vi "Read_Data_Coils.vi"(8 "error in (no error)":errorcluster, 11 "Device in":refnum<class "RS232_Device.lvclass">) -> (0 "error out":errorcluster, 2 "Discrete Inputs":bool[](array[boolean]), 3 "Device out":refnum<class "RS232_Device.lvclass">)   [LabVIEW 2023, in "RS232_Device.lvclass"]
uses:
  RS232_Device.lvclass
  D:/SamparkProdLine/subVIs/DAQ Device/Modbus_Device/DAQ_Device.lvclass
  RS232_Device.lvclass/RS232_Device.ctl
panel:
  out "resulting string":string
  out "Response":string
  out "return count":u32
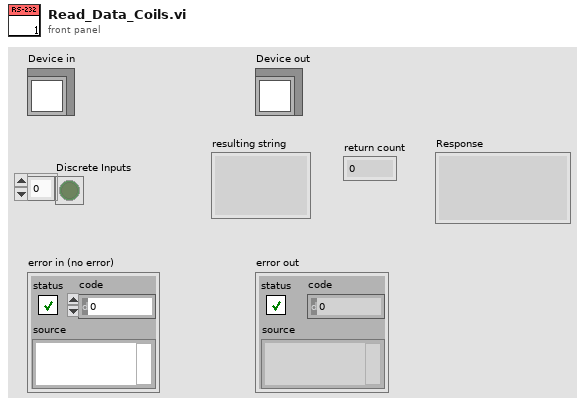
[diagram p1: front panel]
types:
  T1 = typedef "DAQ Device_IO ChannelsData.ctl" = cluster{"#DigitalInputs":u16, "StartAddress_DI":u16, "#DigitalOutputs":u16, "StartAddress_DO":u16, "#AnalogInputs":u16, "StartAddress_AI":u16, "#AnalogOutputs":u16, "StartAddress_AO":u16, "Coil_ReadData":bool[], "Coil_WriteData":bool[], "AI_Data":u16[], "AO_Data":u16[]}
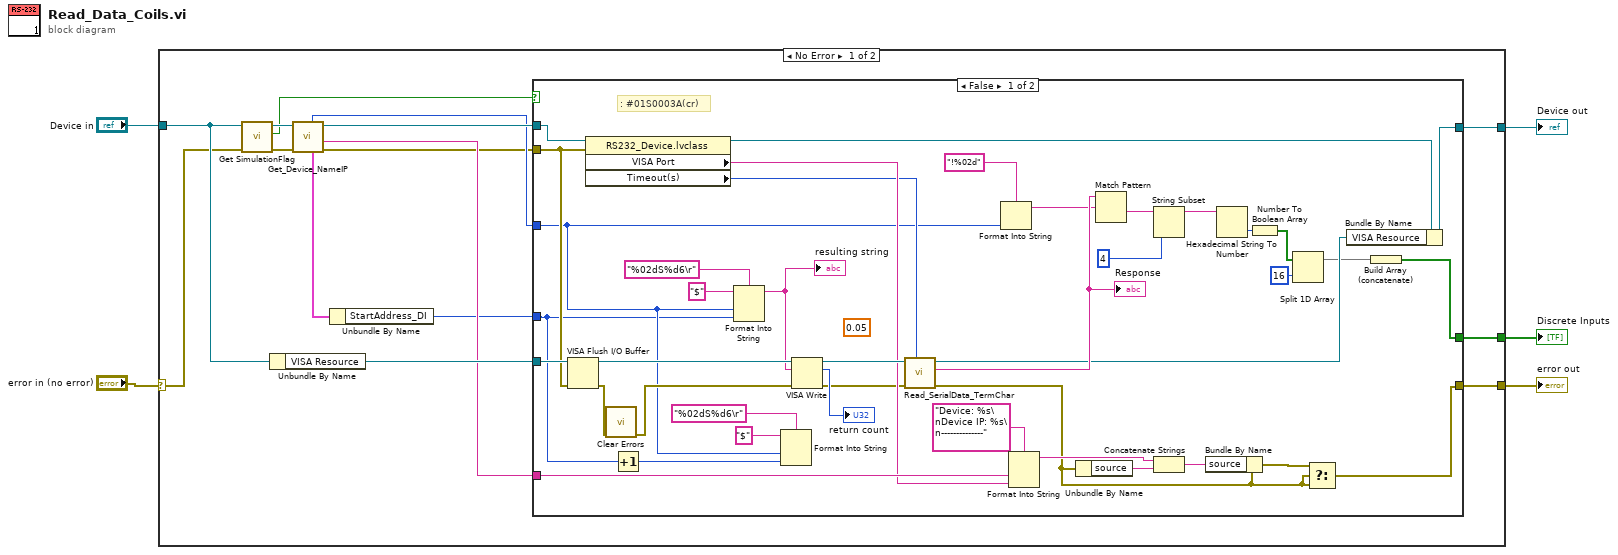
[diagram p0: block diagram]
diagram:
  n1 = case shown="No Error" "error in (no error)" {
    selector: "error in (no error)" -> [w8 w65]
    tunnel: [w19 w65] -> w1
    tunnel: [w20 w64] -> w2
    tunnel: "Device in" -> [w12 w64]
    tunnel: [w17 _] -> w3
    frame No Error {
      n2 = call-dynamic "Get SimulationFlag.vi"("error in (no error)"=w8, "Device in"=w12) -> ("error out"=w16:errorcluster, "Simulation?"=w9:bool, "Device out"=w13:refnum<class "RS232_Device.lvclass">)  [unwired: 7 in]
      n3 = Unbundle By Name(w12) -> ("VISA Resource"=w18:refnum<visa-resource-name>)
      n4 = call-dynamic "Get_Device_NameIP.vi"("error in (no error)"=w16, "Device in"=w13) -> ("error out"=w7:errorcluster, "Device Name"=w10:string, "Device out"=w14:refnum<class "RS232_Device.lvclass">, "IO Channels"=w15:T1, "Unit ID"=w11:u8)  [unwired: 4 in, 1 out]
      n5 = Unbundle By Name(w15) -> ("StartAddress_DI"=w6:u16)
      n6 = case shown="False" w9 {
        tunnel: [w61 w63] -> w20
        tunnel: [w60 w62] -> w19
        tunnel: w18 -> [w59 _]
        tunnel: w14 -> [w41 w63]
        tunnel: w10 -> [w58 _]
        tunnel: [w23 _] -> w17
        tunnel: w11 -> [w30 _]
        tunnel: w6 -> [w29 _]
        tunnel: w7 -> [w40 w62]
        frame False {
          (unwired) 0.05 ("Delay Time (s)")
          # ": #01S0003A(cr)"
          n7 = VISA Flush I/O Buffer(VISA resource name=w59, error in (no error)=w40) -> (VISA resource name out=w52:refnum<visa-resource-name>, error out=w51:errorcluster)  [unwired: 1 in]
          n8 = property class="RS232_Device.lvclass"(reference=w41, error in=w40) -> (reference out=w42:refnum<class "RS232_Device.lvclass">, "VISA Port"=w39:string, "Timeout(s)"=w33:i32)  [unwired: 1 out]
          n9 = call <vilib>:"Clear Errors.vi"("error in (no error)"=w51) -> ("error out"=w50:errorcluster)  [unwired: 5 in, 1 out]
          n10 = Increment(x=w29) -> (x+1=w28:u16)
          n11 = Format Into String(format string="%02dS%d6\r", initial string="$", w30, w29) -> (resulting string=w44:string)  [unwired: 1 in, 1 out]
          "resulting string" <- w44
          n12 = Format Into String(format string="%02dS%d6\r", initial string="$", w30, w28) -> ()  [unwired: 1 in, 2 out]
          n13 = VISA Write(VISA resource name=w52, write buffer=w44, error in (no error)=w50) -> (VISA resource name out=w49:refnum<visa-resource-name>, return count=→"return count":u32, error out=w35:errorcluster)
          n14 = call "Read_SerialData_TermChar.vi"("timeout (50ms)"=w33, "error in (no error)"=w35, "VISA Refnum in"=w49) -> ("error out"=w48:errorcluster, "StringData"=w37:string, "VISA Refnum out"=w34:refnum<visa-resource-name>)  [unwired: 6 in]
          "Response" <- w37
          n15 = Format Into String(format string="!%02d" ("regular expression"), w30) -> (resulting string=w27:string)  [unwired: 2 in, 1 out]
          n16 = Format Into String(format string="Device: %s\nDevice IP: %s\n--------------", w58, w39) -> (resulting string=w54:string)  [unwired: 2 in, 1 out]
          n17 = Unbundle By Name(w48) -> ("source"=w56:string)
          n18 = Match Pattern(string=w37, regular expression=w27) -> (after substring=w38:string)  [unwired: 1 in, 3 out]
          n19 = String Subset(string=w38, length (rest)=4 ("length (rest)")) -> (substring=w22:string)  [unwired: 1 in]
          n20 = Concatenate Strings(w54, w56) -> (w53:string)
          n21 = Bundle By Name(cluster=w48, "source"=w53) -> (w57:errorcluster)
          n22 = Hexadecimal String To Number(string=w22) -> (number=w47:u32)  [unwired: 2 in, 1 out]
          n23 = Number To Boolean Array(number=w47) -> (Boolean array=w25:bool[])
          n24 = Split 1D Array(array=w25, index=16) -> (first subarray=w24:bool[])  [unwired: 1 out]
          n25 = Select(t=w57, s=w48, f=w48) -> (s? t:f=w60:errorcluster)
          n26 = Bundle By Name(cluster=w42, "VISA Resource"=w34) -> (w61:refnum<class "RS232_Device.lvclass">)
          n27 = Build Array (concatenate)(w24) -> (w23:bool[])
        }
        frame True {
        }
      }
    }
    frame Error {
    }
  }
  "error out" <- w1
  "Device out" <- w2
  "Discrete Inputs" <- w3
